vi "Read Response.vi"(8 "error in (no error)":errorcluster, 10 "Commands":T1, 11 "ESM303 in":refnum<class "ESM303.lvclass">) -> (0 "error out":errorcluster, 3 "ESM303 out":refnum<class "ESM303.lvclass">)   [LabVIEW 2018, in "ESM303.lvlib" / "ESM303.lvclass"]
uses:
  ESM303.lvclass
  builds/Force Test Stand.lvlibp/Custom Controls/Commands.ctl
  ESM303.lvclass/ESM303.ctl
  builds/Force Test Stand.lvlibp/Force Test Stand.lvclass
  C:/Users/Ron.Dexter.LUMINARTECH/Desktop/builds/Force Test Stand.lvlibp/Force Test Stand.lvclass
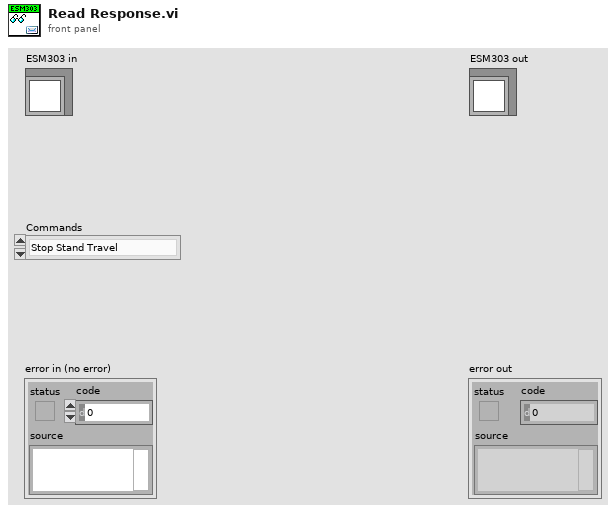
[diagram p1: front panel]
types:
  T1 = typedef "Force Test Stand.lvlibp/Force Test Stand.lvclass/Commands.ctl" = enum16{"Stop Stand Travel", "Start Travel Down (Left)", "Start Travel Up (Right)", "Get Travel Upper Limit", "Get Travel Lower Limit", "Set Travel Upper Limit", "Set Travel Lower Limit", "Get Travel Value", "Set Travel Units (mm)", "Set Travel Units (in)", "Reset Travel to Zero", "Get Speed ", "Set Speed", "Set Speed to Min", "Set Speed to Max", "Get Force Value", "Get Force Units", "Set Force Units (lbF)", "Get Stand Status", "Set Cycle Mode", "Set Limit Mode", "Set Manual Mode", "Set No. Cycles", "Get Travel/Force Values", "Get Completed Cycles", "Get Cycles Setpoint", "Reset Cycles Counter", "Zero Force Gauge", "Set Force Upper Limit", "Set Force Lower Limit", "Get Travel Units", "Get Speed Units", "Default", "Set Force Units (N)", "Set Force Units (kgF)", "Set Force Units (ozF)", "Set Force Units (gF)", "Set Force Real Time Mode", "Set Force Peak Tension Mode", "Set Force Peak Compression Mode", "Set Force High Set-Point", "Set Force Low Set-Point", "Gauge Transmit with Units", "Gauge Transmit w/o Units", "Get Peak Compression Force", "Get Peak Tension Force", "Get Real Time Force", "Disable Force High Limit", "Disable Force Low Limit", "Send Speed Setting to Stand"}
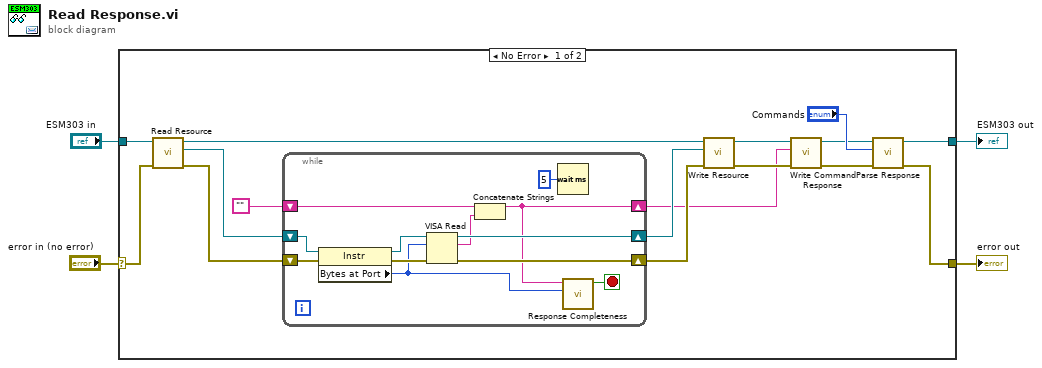
[diagram p0: block diagram]
diagram:
  n1 = case shown="No Error" "error in (no error)" {
    selector: "error in (no error)" -> [w9 w34]
    tunnel: [w10 w34] -> w3
    tunnel: [w5 w33] -> w2
    tunnel: "ESM303 in" -> [w20 w33]
    frame No Error {
      n2 = call "Read Resource.vi"("error in (no error)"=w9, "Force Test Stand in"=w20) -> ("error out"=w19:errorcluster, "Resource"=w18:refnum<visa-resource-name>, "Force Test Stand out"=w17:refnum<class "ESM303.lvclass">)  [unwired: 7 in]
      n3 = while {
        shift-right: [w27] -> w15
        shift-left: w19 -> [w32]
        shift-right: [w28] -> w16
        shift-left: w18 -> [w31]
        shift-right: [w23] -> w7
        shift-left: "" -> [w26]
        stop <- w21 stop-if-true
        n4 = property class="Instr"(reference=w31, error in=w32) -> (reference out=w30:refnum<visa-resource-name>, error out=w29:errorcluster, "Bytes at Port"=w22:u32)
        n5 = VISA Read(VISA resource name=w30, byte count=w22, error in (no error)=w29) -> (VISA resource name out=w28:refnum<visa-resource-name>, read buffer=w25:string, error out=w27:errorcluster)  [unwired: 1 out]
        n6 = Concatenate Strings(w26, w25) -> (w23:string)
        n7 = Wait (ms)(milliseconds to wait=u32 5) -> ()  [unwired: 1 out]
        n8 = call "Response Completeness.vi"("Bytes at Port"=w22, "Response Buffer"=w23) -> ("Response Complete?"=w21:bool)  [unwired: 8 in, 1 out]
      }
      n9 = call "Write Resource.vi"("error in (no error)"=w15, "Resource"=w16, "Force Test Stand in"=w17) -> ("error out"=w13:errorcluster, "Force Test Stand out"=w14:refnum<class "ESM303.lvclass">)  [unwired: 7 in]
      n10 = call "Write Command Response.vi"("error in (no error)"=w13, "Command Response"=w7, "ESM303 in"=w14) -> ("error out"=w11:errorcluster, "ESM303 out"=w6:refnum<class "ESM303.lvclass">)  [unwired: 7 in]
      n11 = call "Parse Response.vi"("error in (no error)"=w11, "Command"="Commands", "ESM303 in"=w6) -> ("error out"=w10:errorcluster, "ESM303 out"=w5:refnum<class "ESM303.lvclass">)  [unwired: 7 in]
    }
    frame Error {
    }
  }
  "error out" <- w3
  "ESM303 out" <- w2
